vi "Python Interoperation Example.vi"() -> ()   [LabVIEW 2020]
uses:
  LabVIEW/g_ar_toolkit.image/CreateEmptyImageARGB.vi
  LabVIEW/g_ar_toolkit.image/CopyArrayToImageARGB.vi
  LabVIEW/g_ar_toolkit.image/DrawImageToPictureARGB.vi
  LabVIEW/g_ar_toolkit.image/CreateEmptyImageARGB.vi/3321fa97-f432-4e1e-8db9-a0df79aed21b.vi
  LabVIEW/g_ar_toolkit.image/CopyArrayToImageARGB.vi/26c70cee-9332-41f4-9755-08948a885cbe.vi
  LabVIEW/g_ar_toolkit.image/DrawImageToPictureARGB.vi/8cd07b1b-062e-4fe4-9e87-2eb3dc89fe0e.vi
  LabVIEW/g_ar_toolkit.image/ARGBColourToU32.vi
  <vilib>/Utility/error.llb/Error Cluster From Error Code.vi
  LabVIEW/g_ar_toolkit.image/g_ar_toolkit.image.lvlib
panel:
  out "error out":errorcluster
  out "Picture":picture
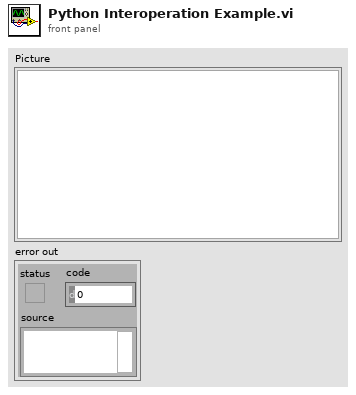
[diagram p1: front panel]
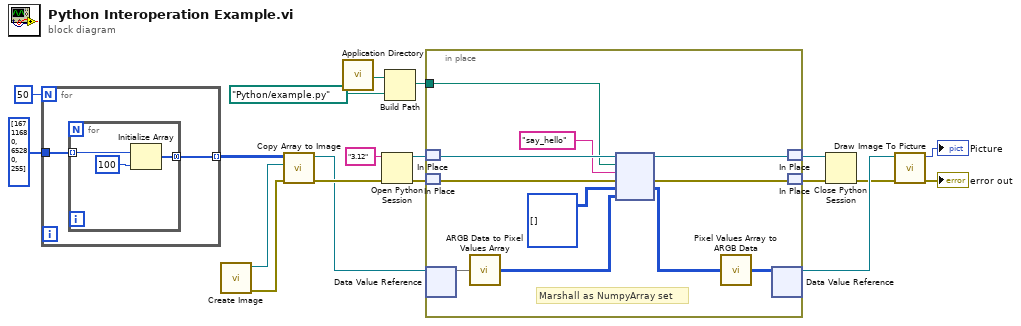
[diagram p0: block diagram]
diagram:
  n1 = for {
    N: 50 -> [_]
    tunnel: u32[] [16711680, 65280, 255] ("color(black)") -> [w21]
    tunnel: [w20] -> w10 mode=indexing
    n2 = for {
      tunnel: w21 -> [w24] mode=indexing
      tunnel: [w22] -> w20 mode=concatenating
      n3 = Initialize Array(w24, 100 ("dimension size")) -> (w22:u32[])
    }
  }
  n4 = call-poly "Create Image.vi"() -> ("error out"=w12:errorcluster, "New ARGB Image"=w11:refnum<data-value>)  [unwired: 10 in]
  n5 = call-poly "Copy Array to Image.vi"("error in (no error)"=w12, "ARGB Image Destination"=w11, "Source"=w10) -> ("error out"=w9:errorcluster, "ARGB Image Destination (Duplicate)"=w6:refnum<data-value>)  [unwired: 7 in]
  n6 = call <vilib>:"Application Directory.vi"() -> ("Application Directory"=w3:path)
  n7 = Open Python Session(python version="3.12" ("Python version"), 3:w9) -> (session out=w17:refnum<k35>, error out=w2:errorcluster)  [unwired: 1 in]
  n8 = Build Path(base path=w3, name or relative path=path "Python/example.py" ("module path")) -> (appended path=w4:path)
  n9 = in-place {
    in-place-border: w4 -> [w27]
    # "Marshall as NumpyArray set"
    n10 = in-place-match #1(w17) -> (w35:refnum<k35>)
    n11 = in-place-match #2(w2) -> (w26:errorcluster)
    n12 = in-place-dvr #3(w6) -> (w32:u32[][])  [unwired: 1 out]
    n13 = call "ARGB Data to Pixel Values Array.vi"("ARGB Data"=w32) -> ("Pixel Values"=w31:u8[][][])
    n14 = node(w35, w27, "say_hello" ("function name"), w26, u8[][][] [] ("Pixel Values"), w31) -> (w34:refnum<k35>, w25:errorcluster, w28:u8[][][])  [unwired: 1 in, 2 out]
    n15 = call "Pixel Values Array to ARGB Data.vi"("Pixel Values"=w28) -> ("ARGB Data"=w30:u32[][])
    n16 = in-place-dvr #3(w30) -> (w14:refnum<data-value>)  [unwired: 1 out]
    n17 = in-place-match #1(w34) -> (w15:refnum<k35>)
    n18 = in-place-match #2(w25) -> (w1:errorcluster)
  }
  n19 = Close Python Session(session in=w15, error in=w1) -> (11:w8:errorcluster)
  n20 = call-poly "Draw Image To Picture.vi"("error in (no error)"=w8, "ARGB Image Source"=w14) -> ("error out"=→"error out":errorcluster, "Picture"=→"Picture":picture)  [unwired: 8 in]
